vi "FTB WPF UDP - Receiver.vi"() -> ()   [LabVIEW 2014]
doc: "The UDP protocol differs from TCP in that there is no error-checking with the packets of information that are sent, and thus no guarantee whatsoever that an intended recipient will actually receive a given piece of data.\n\nUDP does offer the ability to \"broadcast\" data across a network--simply specify an IP Address of all ones (255.255.255.255) to attempt to broadcast information network-wide. Keep in mind that routers and other network hardware will generally refuse to forward the broadcast beyond certain points, so the extent of the broadcast will in practice be limited."
panel:
  out "Coord":sgl
  in  "Stop":bool
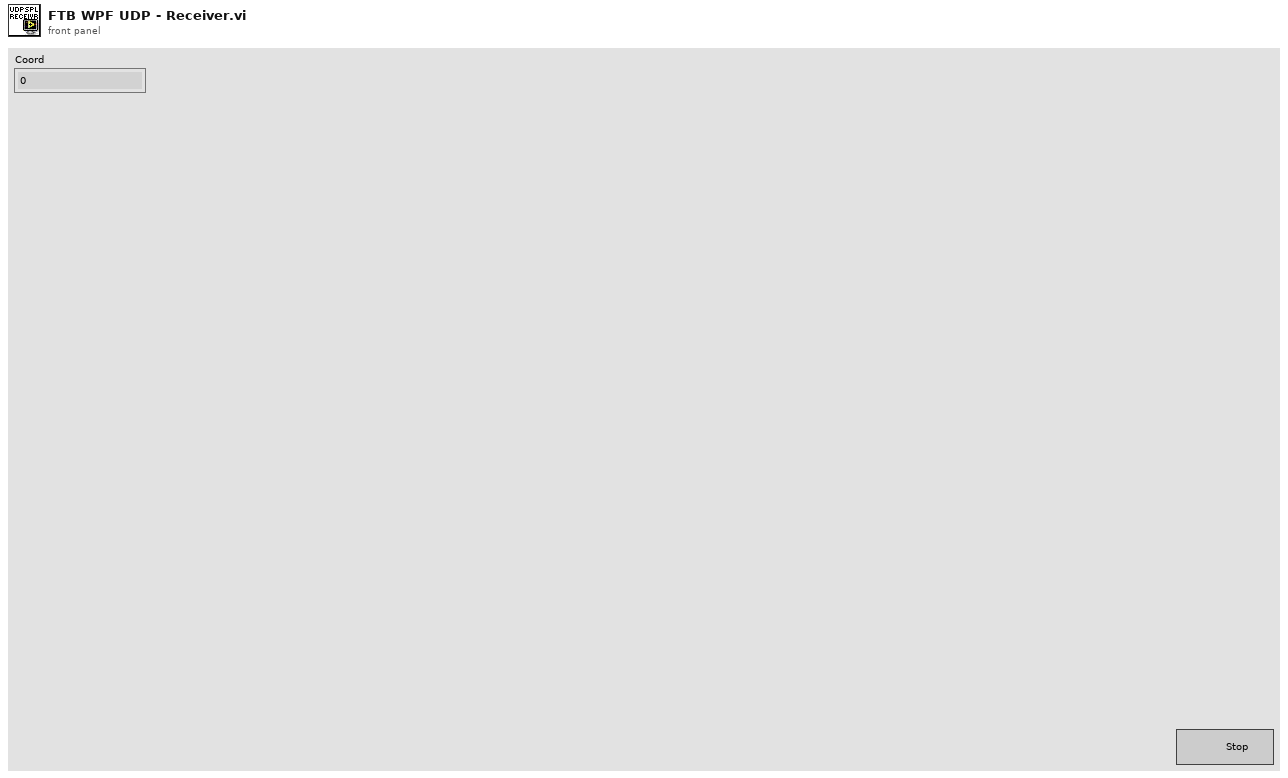
[diagram p1: front panel]
types:
  T1 = enum16{"big-endian, network order", "native, host order", "little-endian"}
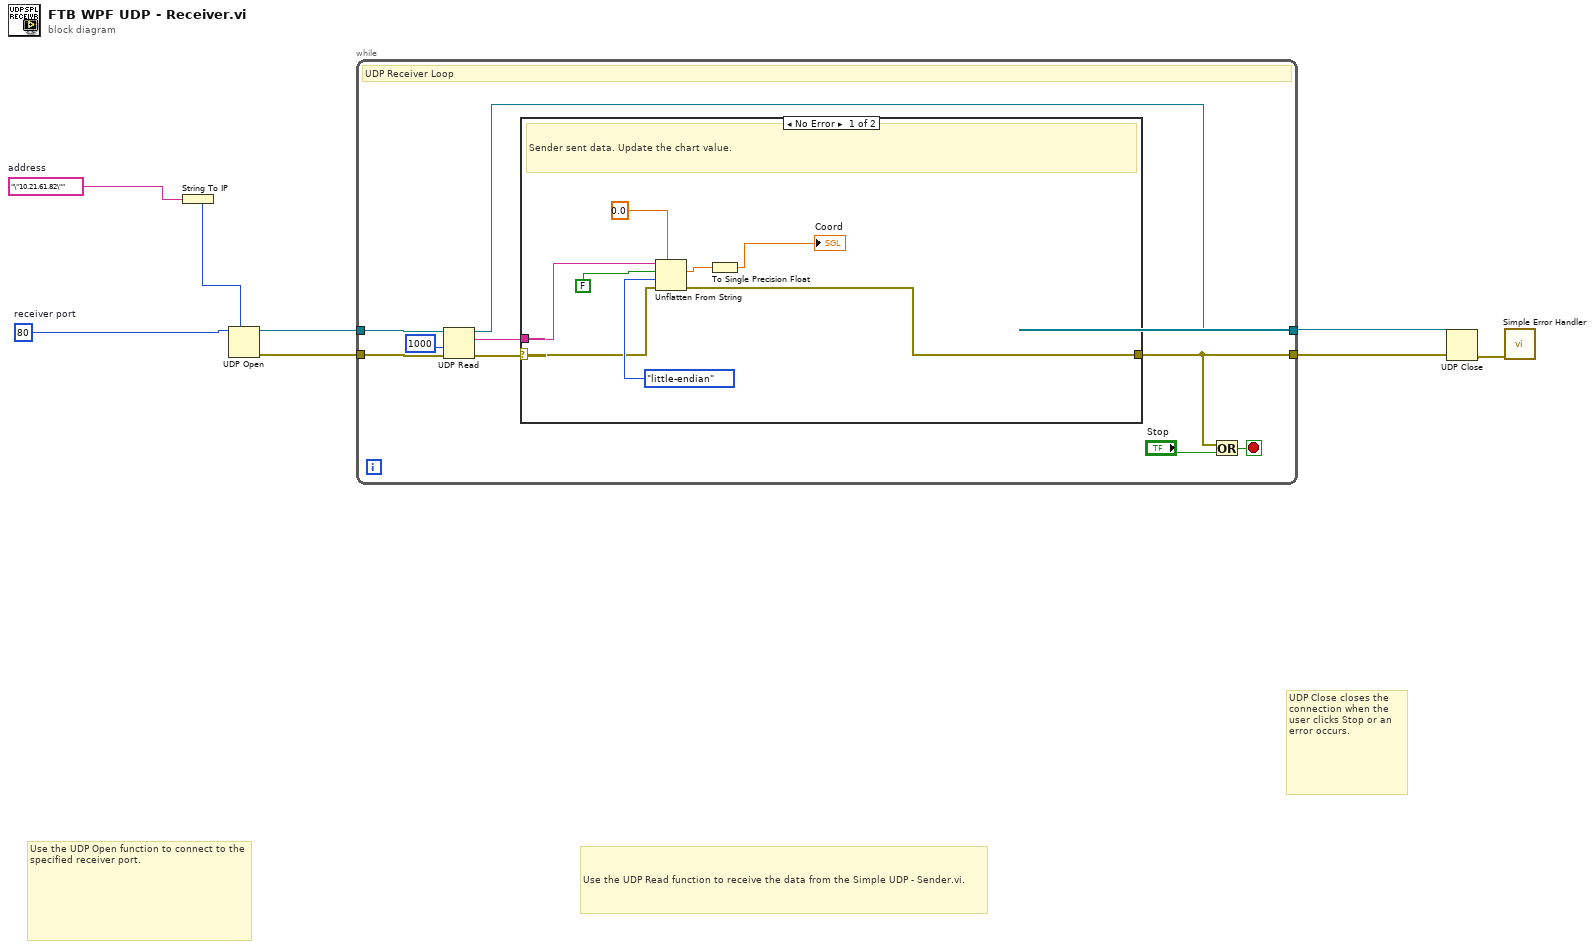
[diagram p0: block diagram]
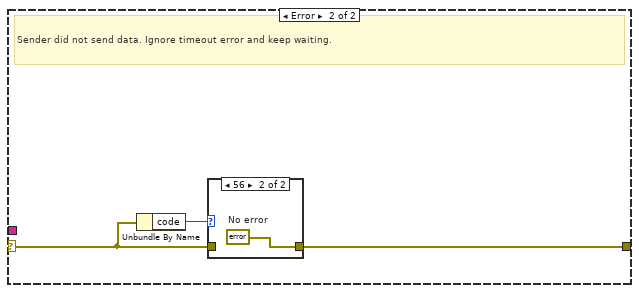
[diagram p2: hidden frame]
diagram:
  w2 = "\"10.21.61.82\""  # address
  w3 = u16 80  # receiver port
  # "UDP Close closes the connection when the user clicks Stop or an error occurs."
  # "Use the UDP Open function to connect to the specified receiver port."
  # "Use the UDP Read function to receive the data from the Simple UDP - Sender.vi."
  n1 = String To IP(1:w2) -> (0:w1:u32)
  n2 = UDP Open(7:w1, 11:w3) -> (port=w4:refnum<k16>, 0:w5:errorcluster)  [unwired: 3 in, 1 out]
  n3 = while {
    tunnel: w4 -> [w17]
    tunnel: [w9] -> w8
    tunnel: w5 -> [w14]
    tunnel: [w10] -> w6
    stop <- w15 stop-if-true
    # "UDP Receiver Loop"
    n4 = UDP Read(connection ID=w17, timeout ms (25000)=1000, 8:w14) -> (data out=w12:string, error out=w11:errorcluster, 3:w9:refnum<k16>)  [unwired: 3 out]
    n5 = case shown="No Error" w11 {
      selector: w11 -> [w22 w27]
      tunnel: w12 -> [w25 _]
      tunnel: [w21 w26] -> w10
      frame No Error {
        # "Sender sent data. Update the chart value."
        n6 = Unflatten From String(type=sgl 0.0, binary string=w25, data includes array or string size? (T)=FALSE, byte order (0:big-endian, network order)=T1."little-endian" ("byte order"), error in (no error)=w22) -> (value=w19:sgl, error out=w21:errorcluster)  [unwired: 1 out]
        n7 = To Single Precision Float(number=w19) -> (single precision float=→"Coord":sgl)
      }
      frame Error {
        # "Sender did not send data. Ignore timeout error and keep waiting."
        n8 = Unbundle By Name(w27) -> ("code"=w28:i32)
        n9 = case shown="56" w28 {
          tunnel: w27 -> [w29 _]
          tunnel: [w29 w30] -> w26
          frame Default {
          }
          frame 56 {
            w30 = errorcluster {"status"=FALSE, "code"=0, "source"=""}  # No error
          }
        }
      }
    }
    n10 = Or(x=w10, y="Stop") -> (x .or. y?=w15:bool)
  }
  n11 = UDP Close(connection ID=w8, 8:w6) -> (error out=w7:errorcluster)  [unwired: 1 out]
  n12 = call <vilib>:"Simple Error Handler.vi"("error in (no error)"=w7) -> ()  [unwired: 1 in, 8 out]
